vi "Init.vi"(6 "JQMHStartup.lvclass":refnum<class "ModuleStartup.lvclass">, 8 "error in (no error)":errorcluster, 10 "Declare? (T)":bool, 11 "JQMHCore.lvclass":refnum<class "Module.lvclass">) -> (0 "error out":errorcluster, 1 "StartupParams":variant, 3 "JQMHCore out":refnum<class "Module.lvclass">, 4 "JQMHStartup out":refnum<class "ModuleStartup.lvclass">, 5 "Event Registration Refnum":refnum<event-registration>, 7 "External Start?":bool)   [LabVIEW 2024, in "ModuleShared.lvlib"]
uses:
  ModuleShared.lvlib
  Startup/ModuleStartup.lvclass
  ModuleCore/Module.lvclass
  Startup/ModuleStartup.lvclass/ModuleStartup.ctl
  ModuleCore/Module.lvclass/Module.ctl
  Watchdog/Watchdog.lvclass
  Startup/Command.ctl
  DebugTrace/DebugTrace.lvlib
  ModuleCore/StopEventArgs.ctl
  ModuleCore/StandardRequests.ctl
  ModuleCore/Show Front Panel--Args.ctl
  ModuleCore/Hide Front Panel.ctl
  ModuleCore/Show Block Diagram.ctl
  ModuleCore/Hide Block Diagram--Args.ctl
  ModuleCore/Reply.ctl
  ModuleCore/InitialiseArgs.ctl
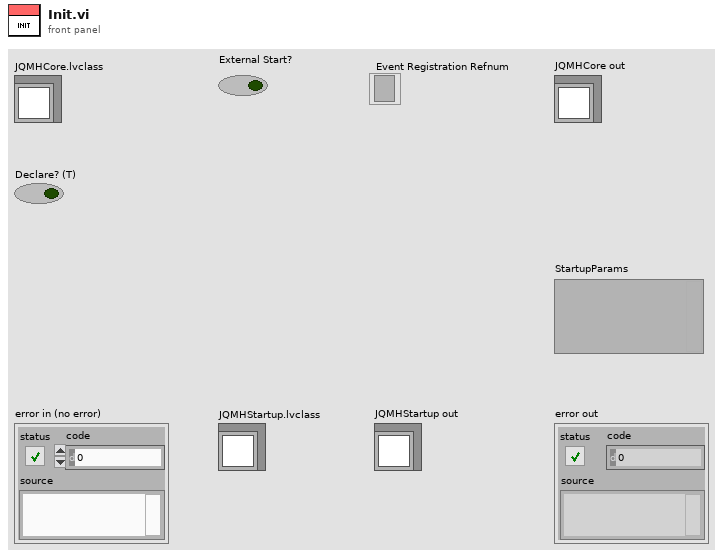
[diagram p1: front panel]
types:
  T1 = typedef "ModuleStartup.lvclass/Command.ctl" = enum16{"Default", "No Override", "Error", "ACK Created", "ACK Mod Reg", "ACK Caller Reg"}
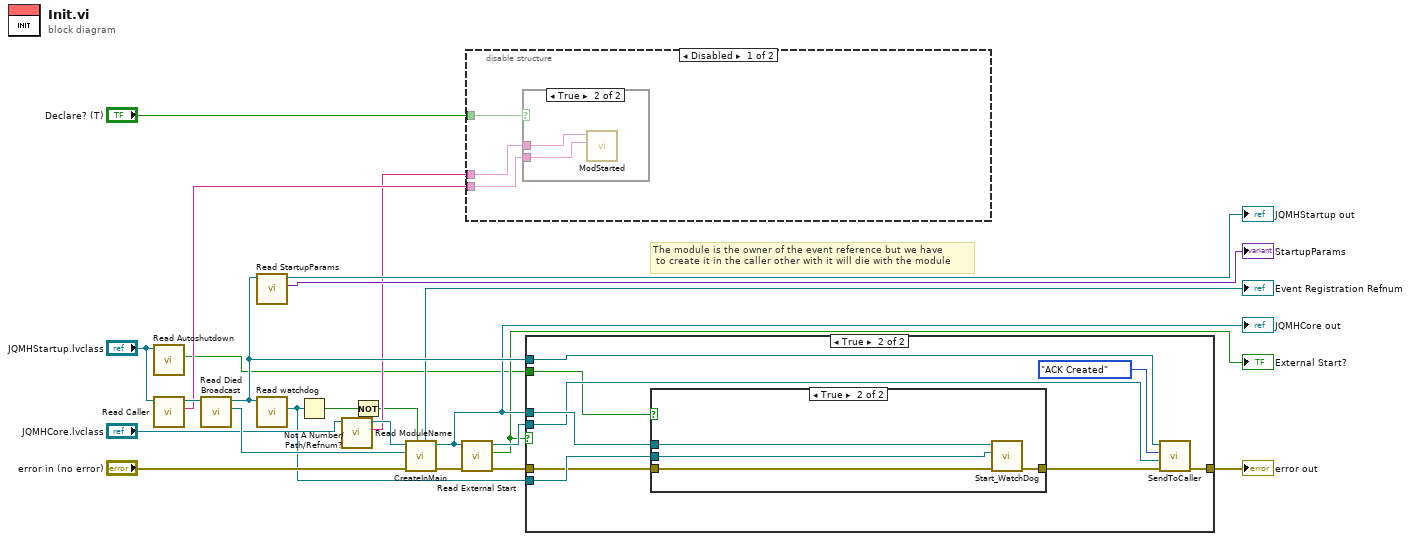
[diagram p0: block diagram]
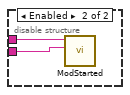
[diagram p3: hidden frame]
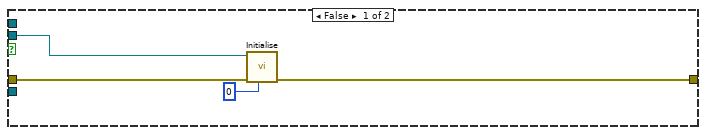
[diagram p4: hidden frame]
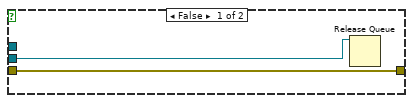
[diagram p5: hidden frame]
diagram:
  # "The module is the owner of the event reference but we have\n to create it in the caller other with it will die with the module"
  n1 = call "Read Autoshutdown.vi"("RQMHStartup in"="JQMHStartup.lvclass") -> ("Autostop?"=w4:bool)  [unwired: 8 in, 2 out]
  n2 = call "Read Caller.vi"("RQMHStartup in"="JQMHStartup.lvclass") -> ("Caller"=w10:string, "RQMHStartup out"=w11:refnum<class "ModuleStartup.lvclass">)  [unwired: 8 in, 1 out]
  n3 = call "Read Died Broadcast.vi"("JQMHStartup in"=w11) -> ("Died Broadcast"=w20:refnum<user-event>, "JQMHStartup out"=w21:refnum<class "ModuleStartup.lvclass">)  [unwired: 9 in]
  n4 = call "Read StartupParams.vi"("JQMHStartup in"=w21) -> ("StartupParams"=→"StartupParams":variant, "JQMHStartup out"=→"JQMHStartup out":refnum<class "ModuleStartup.lvclass">)  [unwired: 8 in, 1 out]
  n5 = call "Read watchdog.vi"("JQMHStartup in"=w21) -> ("watchdog"=w3:refnum<queue>)  [unwired: 8 in, 2 out]
  n6 = Not A Number/Path/Refnum?(number/path/refnum=w3) -> (NaN/Path/Refnum?=w2:bool)
  n7 = call "Read ModuleName.vi"("JQMHModule in"="JQMHCore.lvclass") -> ("ModuleName"=w7:string, "JQMHModule out"=w8:refnum<class "Module.lvclass">)  [unwired: 8 in, 1 out]
  n8 = Not(x=w2) -> (.not. x?=w1:bool)
  n9 = call "CreateInMain.vi"("External Start?"=w1, "error in (no error)"="error in (no error)", "Broadcasts.Died"=w20, "JQMHModule in"=w8) -> ("error out"=w14:errorcluster, "JQMHModule out"=w16:refnum<class "Module.lvclass">, "Event Registration Refnum"=→"Event Registration Refnum":refnum<event-registration>)  [unwired: 5 in]
  "JQMHCore out" <- w16
  n10 = call "Read External Start.vi"("error in (no error)"=w14, "JQMHModule in"=w16) -> ("error out"=w13:errorcluster, "External Start?"=w12:bool, "JQMHModule out"=w15:refnum<class "Module.lvclass">)  [unwired: 7 in]
  "External Start?" <- w12
  n11 = disable-structure shown="Disabled" {
    disable-tunnel: w10 -> [w26 w29]
    disable-tunnel: w7 -> [w25 w30]
    disable-tunnel: "Declare? (T)" -> [w24 _]
    frame Disabled {
      n12 = case shown="True" w24 {
        tunnel: w26 -> [_ w28]
        tunnel: w25 -> [_ w27]
        frame False {
        }
        frame True {
          n13 = call "ModStarted.vi"("Caller"=w28, "Alias"=w27) -> ()  [unwired: 10 in]
        }
      }
    }
    frame Enabled {
      n14 = call "ModStarted.vi"("Caller"=w29, "Alias"=w30) -> ()  [unwired: 10 in]
    }
  }
  n15 = case shown="True" w12 {
    tunnel: w3 -> [_ w43]
    tunnel: w21 -> [_ w42]
    tunnel: [w32 w40] -> w19
    tunnel: w13 -> [w31 w39]
    tunnel: w16 -> [_ w37]
    tunnel: w15 -> [w33 w36]
    tunnel: w4 -> [_ w35]
    frame False {
      n16 = call "Initialise.vi"("timeout in ms (-1)"=0, "error in (no error)"=w31, "JQMHModule in"=w33) -> ("error out"=w32:errorcluster)  [unwired: 5 in, 3 out]
    }
    frame True {
      n17 = case shown="True" w35 {
        tunnel: w37 -> [_ w47]
        tunnel: w43 -> [w44 w46]
        tunnel: w39 -> [w45 w49]
        tunnel: [w45 w48] -> w38
        frame False {
          n18 = Release Queue(queue=w44) -> ()  [unwired: 2 in, 3 out]
        }
        frame True {
          n19 = call "Start_WatchDog.vi"("error in (no error)"=w49, "Caller"=w46, "ModToWatch"=w47) -> ("error out"=w48:errorcluster)  [unwired: 8 in]
        }
      }
      n20 = call "SendToCaller.vi"("error in (no error)"=w38, "Data"=w36, "Command"=Command."ACK Created", "JQMHStartup in"=w42) -> ("error out"=w40:errorcluster)  [unwired: 6 in, 1 out]
    }
  }
  "error out" <- w19
